vi "Manufacturer Identifyer.vi"(11 "Visa In":string) -> (2 "Boolean":bool, 3 "string":string)   [LabVIEW 2016, in "Universal Power Meter.lvlib" / "Universal Power Meter.lvclass"]
uses:
  Universal Power Meter.lvclass
  Manufacturer List.ctl
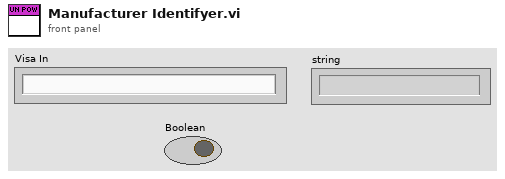
[diagram p1: front panel]
types:
  T1 = typedef "Manufacturer List.ctl" = enum16{"NATIONAL INSTRUMENTS", "TEKTRONIX", "FLUKE", "dummy", "LUTRON", "YOKOGAWA"}
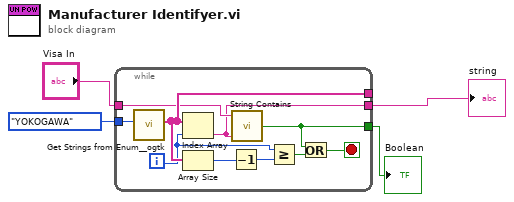
[diagram p0: block diagram]
diagram:
  n1 = while {
    tunnel: Manufacturer_List."YOKOGAWA" ("Manufacturer") -> [w14]
    tunnel: [w13] -> _
    tunnel: "Visa In" -> [w9]
    tunnel: [w5] -> w3
    tunnel: [w6] -> w4
    i -> [w12]
    stop <- w7 stop-if-true
    n2 = call <userlib>:"Get Strings from Enum__ogtk.vi"("Enum"=w14) -> ("Enum Strings"=w13:string[])  [unwired: 7 in, 3 out]
    n3 = Index Array(array=w13, index=w12) -> (element=w6:string)
    n4 = Array Size(array=w13) -> (size(s)=w11:i32)
    n5 = Decrement(x=w11) -> (x-1=w10:i32)
    n6 = call "String Contains.vi"("Regular expression"=w6, "Input String"=w9) -> ("Found?"=w5:bool)  [unwired: 2 in, 1 out]
    n7 = Greater Or Equal?(x=w12, y=w10) -> (x >= y?=w8:bool)
    n8 = Or(x=w5, y=w8) -> (x .or. y?=w7:bool)
  }
  "string" <- w4
  "Boolean" <- w3
